vi "GetTerms4.vi"(0 "XRef":T11, 1 "State In":T10={"Type"=variant(bool FALSE)}) -> (14 "Terms":T2, 15 "Fatal Error Out":T1)   [LabVIEW 2017, in "ReadTag.xnode"]
doc: "Read Tag XNode script that describes the node's connector pane terminals, including their names, types, bounds and directions."
uses:
  ReadTag.xnode
  <vilib>/XNodeSupport/XNodeXNodeRef.ctl
  State.ctl
  <vilib>/XNodeSupport/XNodeTerm4Array.ctl
  <vilib>/XNodeSupport/XNodeTerm4.ctl
  <vilib>/XNodeSupport/XNodeString.ctl
  <vilib>/XNodeSupport/XNodeVariant.ctl
  <vilib>/XNodeSupport/XNodeRect32.ctl
  <vilib>/XNodeSupport/XNodeInt.ctl
  <vilib>/XNodeSupport/XNodeBool.ctl
  <vilib>/XNodeSupport/XNodeTermDirection.ctl
  <vilib>/XNodeSupport/XNodeErrorCluster.ctl
  <vilib>/XNodeSupport/NI_XNodeSupport.lvlib
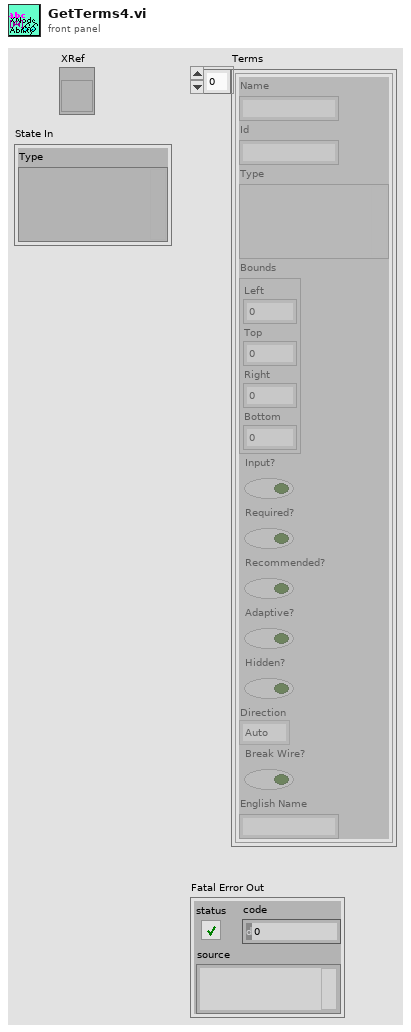
[diagram p1: front panel]
types:
  T1 = typedef "NI_XNodeSupport.lvlib/XNodeErrorCluster.ctl" = errorcluster
  T2 = typedef "NI_XNodeSupport.lvlib/XNodeTerm4Array.ctl" = T3[]
  T3 = typedef "NI_XNodeSupport.lvlib/XNodeTerm4.ctl" = cluster{"Name":T4, "Id":T4, "Type":T5, "Bounds":T6, "Input?":T8, "Required?":T8, "Recommended?":T8, "Adaptive?":T8, "Hidden?":T8, "Direction":T9, "Break Wire?":T8, "English Name":T4}
  T4 = typedef "NI_XNodeSupport.lvlib/XNodeString.ctl" = string
  T5 = typedef "NI_XNodeSupport.lvlib/XNodeVariant.ctl" = variant
  T6 = typedef "NI_XNodeSupport.lvlib/XNodeRect32.ctl" = cluster{"Left":T7, "Top":T7, "Right":T7, "Bottom":T7}
  T7 = typedef "NI_XNodeSupport.lvlib/XNodeInt.ctl" = i32
  T8 = typedef "NI_XNodeSupport.lvlib/XNodeBool.ctl" = bool
  T9 = typedef "NI_XNodeSupport.lvlib/XNodeTermDirection.ctl" = enum32{"Auto", "Up", "Down", "Left", "Right", "Center"}
  T10 = typedef "ReadTag.xnode/State.ctl" = cluster{"Type":variant}
  T11 = typedef "NI_XNodeSupport.lvlib/XNodeXNodeRef.ctl" = refnum<vi>
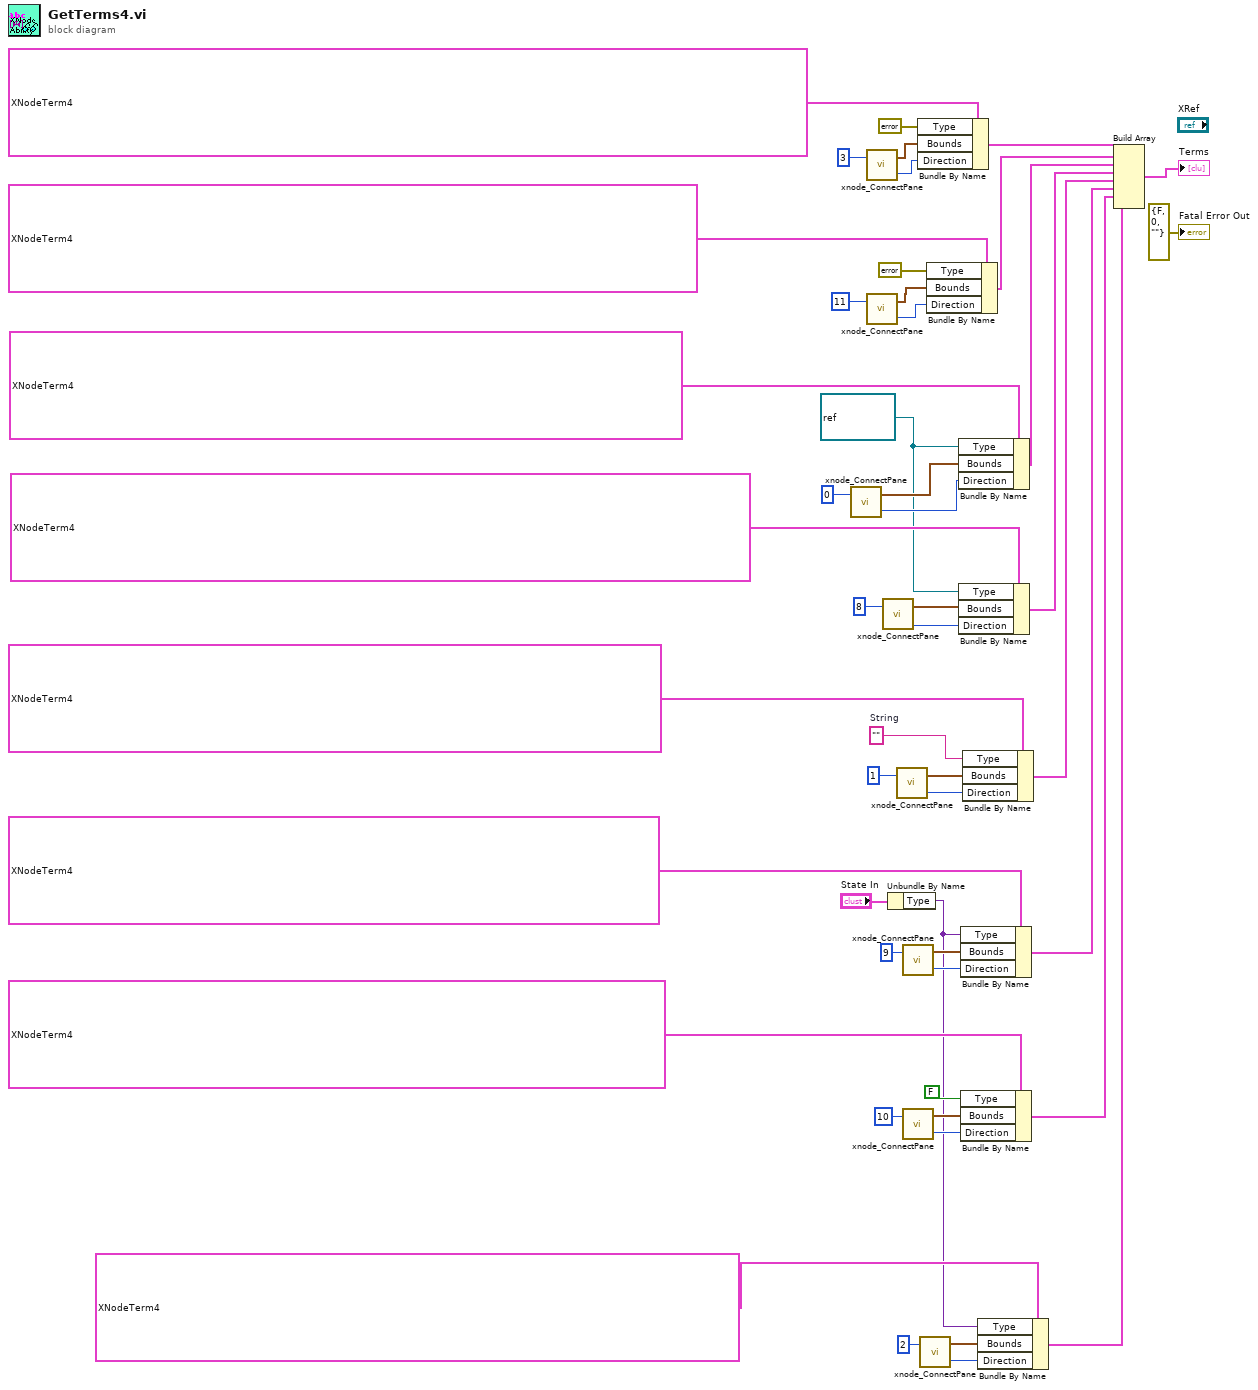
[diagram p0: block diagram]
diagram:
  w19 = ""  # String
  w31 = refnum<data-value> refnum ("data value reference")
  n1 = call "xnode_ConnectPane.vi"("index"=0) -> ("Direction"=w35:T9, "Bounds"=w43:T6)  [unwired: 1 in]
  n2 = call "xnode_ConnectPane.vi"("index"=3) -> ("Direction"=w32:T9, "Bounds"=w38:T6)  [unwired: 1 in]
  n3 = call "xnode_ConnectPane.vi"("index"=11) -> ("Direction"=w33:T9, "Bounds"=w36:T6)  [unwired: 1 in]
  n4 = call "xnode_ConnectPane.vi"("index"=8) -> ("Direction"=w34:T9, "Bounds"=w40:T6)  [unwired: 1 in]
  n5 = Unbundle By Name("State In") -> ("Type"=w2:variant)
  n6 = call "xnode_ConnectPane.vi"("index"=1) -> ("Direction"=w24:T9, "Bounds"=w23:T6)  [unwired: 1 in]
  n7 = call "xnode_ConnectPane.vi"("index"=9) -> ("Direction"=w15:T9, "Bounds"=w18:T6)  [unwired: 1 in]
  n8 = call "xnode_ConnectPane.vi"("index"=10) -> ("Direction"=w12:T9, "Bounds"=w9:T6)  [unwired: 1 in]
  n9 = Bundle By Name(cluster=T3 {"Name"="error in (no error)", "Id"="error in (no error)", "Type"=variant, "Bounds"={"Left"=0, "Top"=24, "Right"=0, "Bottom"=32}, "Input?"=TRUE, "Required?"=FALSE, "Recommended?"=TRUE, "Adaptive?"=FALSE, "Hidden?"=FALSE, "Direction"=enum."Left", "Break Wire?"=FALSE, "English Name"="error in (no error)"} ("Term 4"), "Type"=errorcluster {"status"=FALSE, "code"=0, "source"=""} ("error constant"), "Bounds"=w38, "Direction"=w32) -> (w30:T3)
  n10 = call "xnode_ConnectPane.vi"("index"=2) -> ("Direction"=w4:T9, "Bounds"=w6:T6)  [unwired: 1 in]
  n11 = Bundle By Name(cluster=T3 {"Name"="error out", "Id"="error out", "Type"=variant, "Bounds"={"Left"=32, "Top"=24, "Right"=32, "Bottom"=32}, "Input?"=FALSE, "Required?"=FALSE, "Recommended?"=TRUE, "Adaptive?"=FALSE, "Hidden?"=FALSE, "Direction"=enum."Right", "Break Wire?"=FALSE, "English Name"="error out"} ("Term 4"), "Type"=errorcluster {"status"=FALSE, "code"=0, "source"=""} ("error constant"), "Bounds"=w36, "Direction"=w33) -> (w29:T3)
  n12 = Bundle By Name(cluster=T3 {"Name"="TagMap", "Id"="TagMap", "Type"=variant, "Bounds"={"Left"=0, "Top"=0, "Right"=8, "Bottom"=8}, "Input?"=TRUE, "Required?"=TRUE, "Recommended?"=FALSE, "Adaptive?"=FALSE, "Hidden?"=FALSE, "Direction"=enum."Left", "Break Wire?"=FALSE, "English Name"="TagMap"} ("Term 4"), "Type"=w31, "Bounds"=w43, "Direction"=w35) -> (w28:T3)
  n13 = Bundle By Name(cluster=T3 {"Name"="TagMap(dup)", "Id"="TagMap(dup)", "Type"=variant, "Bounds"={"Left"=0, "Top"=0, "Right"=32, "Bottom"=8}, "Input?"=FALSE, "Required?"=FALSE, "Recommended?"=TRUE, "Adaptive?"=FALSE, "Hidden?"=FALSE, "Direction"=enum."Right", "Break Wire?"=FALSE, "English Name"="TagMap(dup)"} ("Term 4"), "Type"=w31, "Bounds"=w40, "Direction"=w34) -> (w27:T3)
  n14 = Bundle By Name(cluster=T3 {"Name"="Value", "Id"="Value", "Type"=variant, "Bounds"={"Left"=0, "Top"=16, "Right"=0, "Bottom"=24}, "Input?"=FALSE, "Required?"=FALSE, "Recommended?"=TRUE, "Adaptive?"=TRUE, "Hidden?"=FALSE, "Direction"=enum."Left", "Break Wire?"=FALSE, "English Name"="Value"} ("Term 4"), "Type"=w2, "Bounds"=w18, "Direction"=w15) -> (w14:T3)
  n15 = Bundle By Name(cluster=T3 {"Name"="found", "Id"="found", "Type"=variant, "Bounds"={"Left"=0, "Top"=16, "Right"=0, "Bottom"=24}, "Input?"=FALSE, "Required?"=FALSE, "Recommended?"=TRUE, "Adaptive?"=FALSE, "Hidden?"=FALSE, "Direction"=enum."Left", "Break Wire?"=FALSE, "English Name"="found"} ("Term 4"), "Type"=FALSE, "Bounds"=w9, "Direction"=w12) -> (w8:T3)
  n16 = Bundle By Name(cluster=T3 {"Name"="name", "Id"="name", "Type"=variant, "Bounds"={"Left"=0, "Top"=8, "Right"=0, "Bottom"=16}, "Input?"=TRUE, "Required?"=TRUE, "Recommended?"=FALSE, "Adaptive?"=FALSE, "Hidden?"=FALSE, "Direction"=enum."Left", "Break Wire?"=FALSE, "English Name"="name"} ("Term 4"), "Type"=w19, "Bounds"=w23, "Direction"=w24) -> (w20:T3)
  n17 = Bundle By Name(cluster=T3 {"Name"="Type", "Id"="Type", "Type"=variant, "Bounds"={"Left"=0, "Top"=8, "Right"=0, "Bottom"=16}, "Input?"=TRUE, "Required?"=TRUE, "Recommended?"=FALSE, "Adaptive?"=TRUE, "Hidden?"=FALSE, "Direction"=enum."Left", "Break Wire?"=FALSE, "English Name"="Type"} ("Term 4"), "Type"=w2, "Bounds"=w6, "Direction"=w4) -> (w1:T3)
  n18 = Build Array(w30, w29, w28, w27, w20, w14, w8, w1) -> (→"Terms":T3[])
  "Fatal Error Out" <- T1 {"status"=FALSE, "code"=0, "source"=""} ("Fatal Error Out")
